vi "SL1.vi"   [LabVIEW 2015, in "Lego_Swerve_2015.lvrbt"]
uses:
  Lego_Swerve_2015.lvrbt
  <vilib>/NXT/Dual Mode Library/BT/BlueTooth_Read_string.vi
  <vilib>/NXT/Dual Mode Library/Display/drawText.vi
types:
  T1 = typedef "LVHSConnector.ctl" = refnum<class "BrickReference.lvclass">
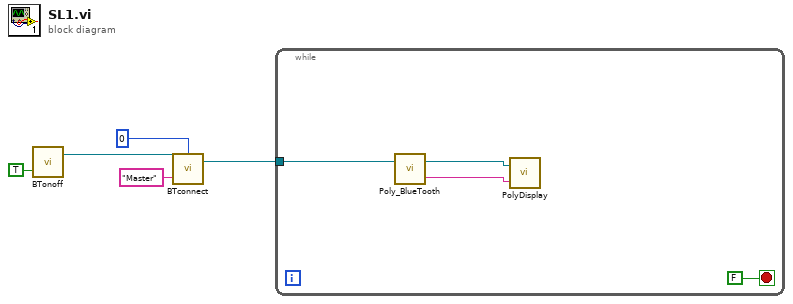
[diagram p0: block diagram]
diagram:
  n1 = call <vilib>:"BTonoff.vi"("On/Off"=TRUE) -> ("NXT/EV3"=w5:T1)  [unwired: 2 in, 1 out]
  n2 = call <vilib>:"BTconnect.vi"("Partner Name"="Master", "NXT/EV3"=w5, "Connection"=u8 0) -> ("NXT/EV3"=w3:T1)  [unwired: 1 out]
  n3 = while {
    tunnel: w3 -> [w8]
    stop <- FALSE stop-if-true
    n4 = call-poly <vilib>:"Poly_BlueTooth.vi"("NXT/EV3"=w8) -> ("Message"=w6:string, "NXT/EV3"=w7:T1)  [unwired: 2 in]
    n5 = call-poly <vilib>:"PolyDisplay.vi"("Text"=w6, "NXT/EV3"=w7) -> ()  [unwired: 2 in, 1 out]
  }
